vi "destroy.vi"(8 "error in":errorcluster, 11 "Nominal Client":refnum<class "Nominal Client.lvclass">) -> (0 "error out":errorcluster)   [LabVIEW 2020, in "Nominal Client.lvclass"]
uses:
  Nominal Client.lvclass
  Nominal Client.lvclass/Nominal Client.ctl
  <vilib>/addons/_JKI.lib/REST Client/classes/REST Client/REST Client.lvclass
  submodules/reqwest-labview/lv-src/reqwest/reqwest.lvclass
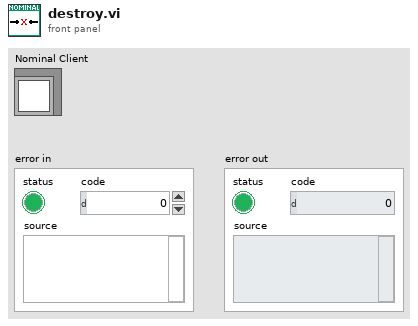
[diagram p1: front panel]
types:
  T1 = typedef "Nominal Client.lvclass/private_data.ctl" = cluster{"API Token":string, "REST Client":refnum<class "REST Client.lvclass">, "workspace":refnum<class "workspace.lvclass">, "Available Workspaces":refnum<class "workspace.lvclass">[], "reqwest":refnum<class "reqwest.lvclass">}
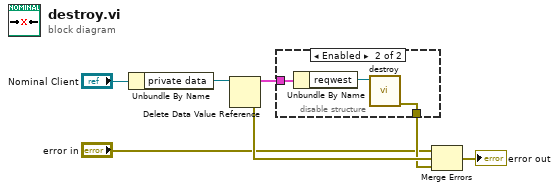
[diagram p0: block diagram]
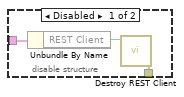
[diagram p2: hidden frame]
diagram:
  n1 = Unbundle By Name("Nominal Client") -> ("private data"=w6:refnum<data-value>)
  n2 = Delete Data Value Reference(data value reference=w6) -> (data value=w5:T1, error out=w4:errorcluster)  [unwired: 1 in]
  n3 = disable-structure shown="Enabled" {
    disable-tunnel: w5 -> [w10 w13]
    disable-tunnel: [w8 w11] -> w3
    frame Disabled {
      n4 = Unbundle By Name(w10) -> ("REST Client"=w9:refnum<class "REST Client.lvclass">)
      n5 = call-dynamic "Destroy REST Client.vi"("REST Client in"=w9) -> ("error out"=w8:errorcluster)  [unwired: 10 in]
    }
    frame Enabled {
      n6 = Unbundle By Name(w13) -> ("reqwest"=w12:refnum<class "reqwest.lvclass">)
      n7 = call "destroy.vi"("reqwest"=w12) -> ("error out"=w11:errorcluster)  [unwired: 10 in]
    }
  }
  n8 = Merge Errors("error in", w4, w3) -> (→"error out":errorcluster)
